vi "VI Tree.vi"   [LabVIEW 2018, in "Fluke 9500B.lvlib"]
doc: "This is the instrument driver for the <INSTRUMENT NAME>. The VI Tree displays all the user-callable VIs of the instrument driver in an organized table."
uses:
  <instrlib>/Fluke 9500B/Fluke 9500B.lvlib
panel:
  # "SEE DIAGRAM\nFOR VI TREE."
  # "MIT License\n\nCopyright (c) 2021 ning\n\nPermission is hereby granted, free of charge, to any person obtaining a copy\nof this software and associated documentation files (the \"Software\"), to deal\nin the Software without restriction, including without limitation the rights\nto use, copy, modify, merge, publish, distribute, sublicense, and/or sell\ncopies of the Software, and to permit persons to whom the Software is\nfurnished to do so, subject to the following conditions:\n\nThe above copyright notice and this permission notice shall be included in all\ncopies or substantial portions of the Software.\n\nTHE SOFTWARE IS PROVIDED \"AS IS\", WITHOUT WARRANTY OF ANY KIND, EXPRESS OR\nIMPLIED, INCLUDING BUT NOT LIMITED TO THE WARRANTIES OF MERCHANTABILITY,\nFITNESS FOR A PARTICULAR PURPOSE AND NONINFRINGEMENT. IN NO EVENT SHALL THE\nAUTHORS OR COPYRIGHT HOLDERS BE LIABLE FOR ANY CLAIM, DAMAGES OR OTHER\nLIABILITY, WHETHER IN AN ACTION OF CONTRACT, TORT OR OTHERWISE, ARISING FROM,\nOUT OF OR IN CONNECTION WITH THE SOFTWARE OR THE USE OR OTHER DEALINGS IN THE\nSOFTWARE."
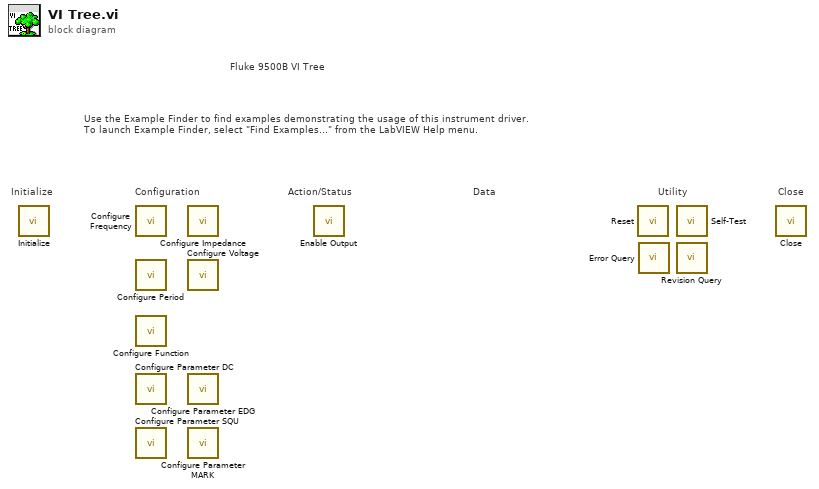
[diagram p0: block diagram]
diagram:
  # "Fluke 9500B VI Tree"
  # "Use the Example Finder to find examples demonstrating the usage of this instrument driver.\nTo launch Example Finder, select \"Find Examples...\" from the LabVIEW Help menu."
  # "Configuration"
  # "Utility"
  # "Data"
  # "Action/Status"
  # "Close"
  # "Initialize"
  n1 = call <instrlib>:"Initialize.vi"() -> ()  [unwired: 10 in, 2 out]
  n2 = call <instrlib>:"Configure Frequency.vi"() -> ()  [unwired: 10 in, 2 out]
  n3 = call <instrlib>:"Configure Period.vi"() -> ()  [unwired: 10 in, 2 out]
  n4 = call <instrlib>:"Configure Function.vi"() -> ()  [unwired: 10 in, 2 out]
  n5 = call <instrlib>:"Configure Parameter DC.vi"() -> ()  [unwired: 12 in]
  n6 = call <instrlib>:"Configure Parameter SQU.vi"() -> ()  [unwired: 10 in, 2 out]
  n7 = call <instrlib>:"Configure Impedance.vi"() -> ()  [unwired: 10 in, 2 out]
  n8 = call <instrlib>:"Configure Voltage.vi"() -> ()  [unwired: 10 in, 2 out]
  n9 = call <instrlib>:"Configure Parameter EDG.vi"() -> ()  [unwired: 10 in, 2 out]
  n10 = call <instrlib>:"Configure Parameter MARK.vi"() -> ()  [unwired: 10 in, 2 out]
  n11 = call <instrlib>:"Enable Output.vi"() -> ()  [unwired: 10 in, 2 out]
  n12 = call <instrlib>:"Reset.vi"() -> ()  [unwired: 10 in, 2 out]
  n13 = call <instrlib>:"Error Query.vi"() -> ()  [unwired: 8 in, 4 out]
  n14 = call <instrlib>:"Self-Test.vi"() -> ()  [unwired: 8 in, 4 out]
  n15 = call <instrlib>:"Revision Query.vi"() -> ()  [unwired: 8 in, 4 out]
  n16 = call <instrlib>:"Close.vi"() -> ()  [unwired: 11 in, 1 out]
